vi "Write Read.vi"(5 "Byte Count":u32, 6 "Timeout ms (1000)":i32=1000, 7 "error in (no error)":errorcluster, 8 "Bytes to Write":u8[](array[numeric]), 9 "Slave Address (7-bit)":u8, 10 "I2C Ref In":T1={"myRIO Reference"={"myRIO Model"=enum."Unknown", "myRIO Hardware Reference"={"Generic FPGA Reference"=refnum, "Allow multiple opens"=FALSE}}, "I2C Channels Enum"=enum."Not Connected", "I2C Configuration"={"I2C Transfer Rate"=enum."Fast mode (400 kbps)"}}) -> (0 "error out":errorcluster, 2 "Bytes Read":u8[](array[numeric]), 3 "I2C Ref Out":T1={"myRIO Reference"={"myRIO Model"=enum."Unknown", "myRIO Hardware Reference"={"Generic FPGA Reference"=refnum, "Allow multiple opens"=FALSE}}, "I2C Channels Enum"=enum."Not Connected", "I2C Configuration"={"I2C Transfer Rate"=enum."Fast mode (400 kbps)"}})   [LabVIEW 2021, in "I2C.lvlib"]
doc: "Writes data to an Inter-Integrated Circuit (I2C) slave device and then reads a specified number of bytes of data from the I2C slave device. This VI returns the result when finishing writing or reading all the bytes, or when timing out."
uses:
  <vilib>/myRIO/Instrument Drivers/Onboard IO/I2C/I2C.lvlib
  <vilib>/myRIO/Instrument Drivers/Onboard IO/I2C/typedefs/I2C Reference.ctl
  <vilib>/myRIO/Common/Instrument Driver Framework/Utilities/typedefs/myRIO Generic Hardware Reference.ctl
  <vilib>/myRIO/Common/Instrument Driver Framework/Utilities/typedefs/Hardware Version Enum.ctl
  <vilib>/myRIO/Common/Instrument Driver Framework/Utilities/typedefs/myRIO v1.0 Reference.ctl
  <vilib>/myRIO/Common/Instrument Driver Framework/Utilities/typedefs/Generic FPGA Reference.ctl
  <vilib>/myRIO/Common/Instrument Driver Framework/myRIO v1.0/I2C/typedefs/I2C Channels Enum.ctl
  <vilib>/myRIO/Instrument Drivers/Onboard IO/I2C/typedefs/I2C Configuration.ctl
  <vilib>/myRIO/Instrument Drivers/Onboard IO/I2C/typedefs/I2C Transfer Rate.ctl
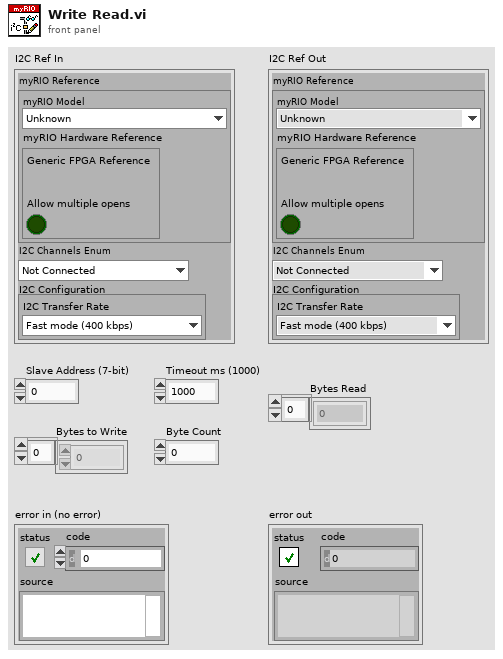
[diagram p1: front panel]
types:
  T1 = typedef "I2C.lvlib/I2C Reference.ctl" = cluster{"myRIO Reference":T2, "I2C Channels Enum":T6, "I2C Configuration":T7}
  T2 = typedef "myRIO Generic Hardware Reference.ctl" = cluster{"myRIO Model":T3, "myRIO Hardware Reference":T4}
  T3 = typedef "Hardware Version Enum.ctl" = enum16{"Unknown", "myRIO-1900", "myRIO-1950", "roboRIO", "NI ELVIS RIO CM", "ELVIS III"}
  T4 = typedef "myRIO v1.0 Reference.ctl" = cluster{"Generic FPGA Reference":T5, "Allow multiple opens":bool}
  T5 = typedef "Generic FPGA Reference.ctl" = refnum<k20>
  T6 = typedef "I2C Channels Enum.ctl" = enum16{"Not Connected", "A/I2C", "B/I2C", "I2C/I2C"}
  T7 = typedef "I2C.lvlib/I2C Configuration.ctl" = cluster{"I2C Transfer Rate":T8}
  T8 = typedef "I2C.lvlib/I2C Transfer Rate.ctl" = enum16{"Standard mode (100 kbps)", "Fast mode (400 kbps)"}
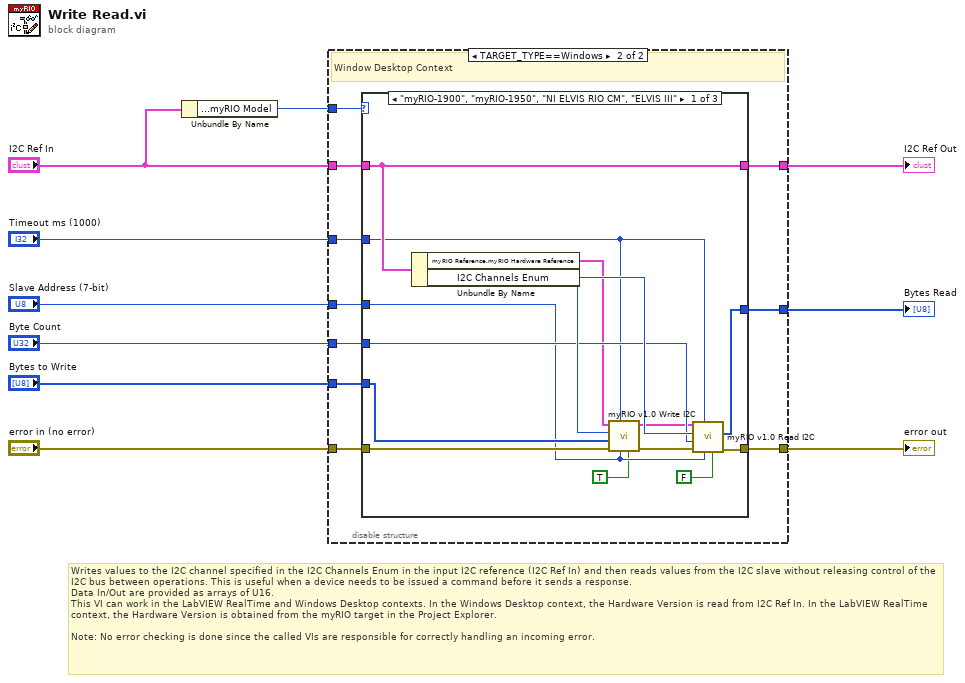
[diagram p0: block diagram]
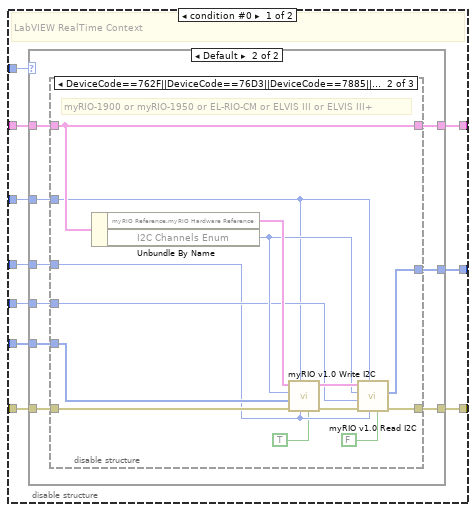
[diagram p2: hidden frame]
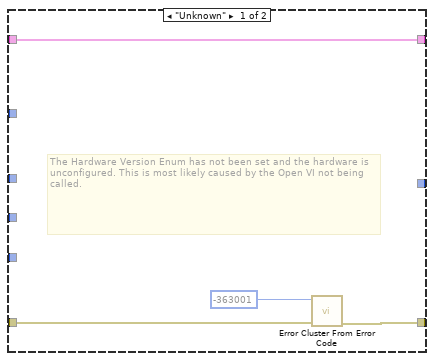
[diagram p3: hidden frame]
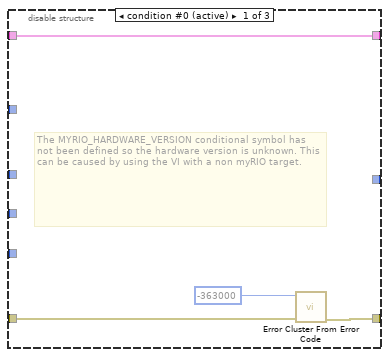
[diagram p4: hidden frame]
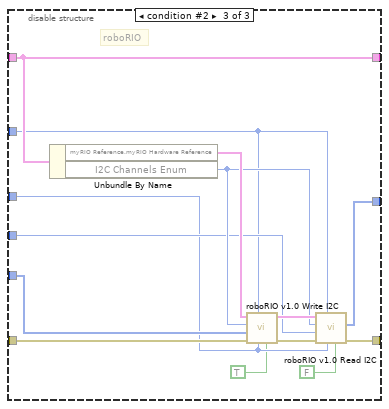
[diagram p5: hidden frame]
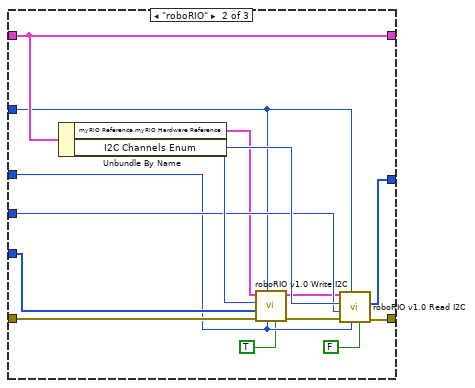
[diagram p6: hidden frame]
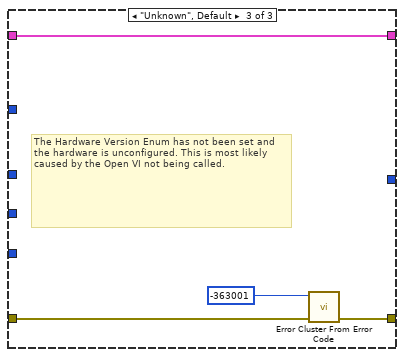
[diagram p7: hidden frame]
diagram:
  # "Writes values to the I2C channel specified in the I2C Channels Enum in the input I2C reference (I2C Ref In) and then reads values from the I2C slave without releasing control of the I2C bus between operations. This is useful when a device needs to be issued a command before it sends a response.\nData In/Out are provided as arrays of U16.\nThis VI can work in the LabVIEW RealTime and Windows Desktop contexts. In the Windows Desktop context, the Hardware Version is read from I2C Ref In. In the LabVIEW RealTime context, the Hardware Version is obtained from the myRIO target in the Project Explorer.\n\nNote: No error checking is done since the called VIs are responsible for correctly handling an incoming error."
  n1 = Unbundle By Name("I2C Ref In") -> ("myRIO Reference.myRIO Model"=w2:T3)
  n2 = disable-structure shown="TARGET_TYPE==Windows" {
    disable-tunnel: [w20 w75] -> w7
    disable-tunnel: "I2C Ref In" -> [w19 w72]
    disable-tunnel: "error in (no error)" -> [w18 w74]
    disable-tunnel: [w17 w73] -> w8
    disable-tunnel: w2 -> [w16 w71]
    disable-tunnel: "Bytes to Write" -> [w15 w70]
    disable-tunnel: "Slave Address (7-bit)" -> [w14 w69]
    disable-tunnel: "Byte Count" -> [w13 w68]
    disable-tunnel: [w12 w67] -> w3
    disable-tunnel: "Timeout ms (1000)" -> [w11 w66]
    frame condition #0 {
      # "LabVIEW RealTime Context"
      n3 = case shown="Default" w16 {
        tunnel: [w23 w33] -> w20
        tunnel: w19 -> [w21 w32]
        tunnel: w18 -> [w22 w31]
        tunnel: [w21 w30] -> w17
        tunnel: w15 -> [_ w29]
        tunnel: w14 -> [_ w28]
        tunnel: w13 -> [_ w27]
        tunnel: [_ w26] -> w12
        tunnel: w11 -> [_ w25]
        frame "Unknown" {
          # "The Hardware Version Enum has not been set and the hardware is unconfigured. This is most likely caused by the Open VI not being called."
          n4 = call <vilib>:"Error Cluster From Error Code.vi"("error in (no error)"=w22, "error code (0)"=-363001) -> ("error out"=w23:errorcluster)  [unwired: 7 in]
        }
        frame Default {
          n5 = disable-structure shown="DeviceCode==762F||DeviceCode==76D3||DeviceCode==7885||DeviceCode==7928||DeviceCode==793C" {
            disable-tunnel: w32 -> [w34 w50 w64]
            disable-tunnel: [w37 w47 w61] -> w33
            disable-tunnel: w31 -> [w35 w49 w63]
            disable-tunnel: [w34 w50 w64] -> w30
            disable-tunnel: w29 -> [_ w48 w62]
            disable-tunnel: w28 -> [_ w42 w56]
            disable-tunnel: w27 -> [_ w43 w57]
            disable-tunnel: [_ w40 w54] -> w26
            disable-tunnel: w25 -> [_ w39 w53]
            frame condition #0 (active) {
              # "The MYRIO_HARDWARE_VERSION conditional symbol has not been defined so the hardware version is unknown. This can be caused by using the VI with a non myRIO target."
              n6 = call <vilib>:"Error Cluster From Error Code.vi"("error in (no error)"=w35, "error code (0)"=-363000) -> ("error out"=w37:errorcluster)  [unwired: 7 in]
            }
            frame condition #1 {
              # "myRIO-1900 or myRIO-1950 or EL-RIO-CM or ELVIS III or ELVIS III+"
              n7 = Unbundle By Name(w50) -> ("myRIO Reference.myRIO Hardware Reference"=w51:T4, "I2C Channels Enum"=w44:T6)
              n8 = call <vilib>:"myRIO v1.0 Write I2C.vi"("Keep Bus Busy"=TRUE ("Generate STOP"), "Slave Address (7-bit)"=w42, "Timeout ms (1000)"=w39, "Error In (No Error)"=w49, "Data to Write"=w48, "Channel"=w44, "myRIO Ref In"=w51) -> ("error out"=w46:errorcluster, "myRIO Ref Out"=w45:T4)  [unwired: 3 in]
              n9 = call <vilib>:"myRIO v1.0 Read I2C.vi"("Keep Bus Busy"=FALSE, "Slave Address (7-bit)"=w42, "Timeout ms (1000)"=w39, "Error In (No Error)"=w46, "Bytes to Read"=w43, "Channel"=w44, "myRIO Ref In"=w45) -> ("error out"=w47:errorcluster, "Data Read"=w40:u8[])  [unwired: 2 in, 1 out]
            }
            frame condition #2 {
              # "roboRIO"
              n10 = Unbundle By Name(w64) -> ("myRIO Reference.myRIO Hardware Reference"=w65:T4, "I2C Channels Enum"=w58:T6)
              n11 = call <vilib>:"roboRIO v1.0 Write I2C.vi"("Keep Bus Busy"=TRUE ("Generate STOP"), "Slave Address (7-bit)"=w56, "Timeout ms (1000)"=w53, "Error In (No Error)"=w63, "Data to Write"=w62, "Channel"=w58, "myRIO Ref In"=w65) -> ("error out"=w60:errorcluster, "myRIO Ref Out"=w59:T4)  [unwired: 3 in]
              n12 = call <vilib>:"roboRIO v1.0 Read I2C.vi"("Keep Bus Busy"=FALSE, "Slave Address (7-bit)"=w56, "Timeout ms (1000)"=w53, "Error In (No Error)"=w60, "Bytes to Read"=w57, "Channel"=w58, "myRIO Ref In"=w59) -> ("error out"=w61:errorcluster, "Data Read"=w54:u8[])  [unwired: 2 in, 1 out]
            }
          }
        }
      }
    }
    frame condition #1 (active) {
      # "Window Desktop Context"
      n13 = case shown="\"myRIO-1900\", \"myRIO-1950\", \"NI ELVIS RIO CM\", \"ELVIS III\"" w71 {
        tunnel: [w80 w94 w107] -> w75
        tunnel: w72 -> [w89 w103 w104]
        tunnel: w74 -> [w88 w102 w105]
        tunnel: [w89 w103 w104] -> w73
        tunnel: w70 -> [w87 w101 _]
        tunnel: w69 -> [w79 w93 _]
        tunnel: w68 -> [w85 w99 _]
        tunnel: [w81 w95 _] -> w67
        tunnel: w66 -> [w77 w91 _]
        frame "myRIO-1900", "myRIO-1950", "NI ELVIS RIO CM", "ELVIS III" {
          n14 = Unbundle By Name(w89) -> ("myRIO Reference.myRIO Hardware Reference"=w83:T4, "I2C Channels Enum"=w86:T6)
          n15 = call <vilib>:"myRIO v1.0 Write I2C.vi"("Keep Bus Busy"=TRUE ("Generate STOP"), "Slave Address (7-bit)"=w79, "Timeout ms (1000)"=w77, "Error In (No Error)"=w88, "Data to Write"=w87, "Channel"=w86, "myRIO Ref In"=w83) -> ("error out"=w84:errorcluster, "myRIO Ref Out"=w82:T4)  [unwired: 3 in]
          n16 = call <vilib>:"myRIO v1.0 Read I2C.vi"("Keep Bus Busy"=FALSE, "Slave Address (7-bit)"=w79, "Timeout ms (1000)"=w77, "Error In (No Error)"=w84, "Bytes to Read"=w85, "Channel"=w86, "myRIO Ref In"=w82) -> ("error out"=w80:errorcluster, "Data Read"=w81:u8[])  [unwired: 2 in, 1 out]
        }
        frame "roboRIO" {
          n17 = Unbundle By Name(w103) -> ("myRIO Reference.myRIO Hardware Reference"=w97:T4, "I2C Channels Enum"=w100:T6)
          n18 = call <vilib>:"roboRIO v1.0 Write I2C.vi"("Keep Bus Busy"=TRUE ("Generate STOP"), "Slave Address (7-bit)"=w93, "Timeout ms (1000)"=w91, "Error In (No Error)"=w102, "Data to Write"=w101, "Channel"=w100, "myRIO Ref In"=w97) -> ("error out"=w98:errorcluster, "myRIO Ref Out"=w96:T4)  [unwired: 3 in]
          n19 = call <vilib>:"roboRIO v1.0 Read I2C.vi"("Keep Bus Busy"=FALSE, "Slave Address (7-bit)"=w93, "Timeout ms (1000)"=w91, "Error In (No Error)"=w98, "Bytes to Read"=w99, "Channel"=w100, "myRIO Ref In"=w96) -> ("error out"=w94:errorcluster, "Data Read"=w95:u8[])  [unwired: 2 in, 1 out]
        }
        frame "Unknown", Default {
          # "The Hardware Version Enum has not been set and the hardware is unconfigured. This is most likely caused by the Open VI not being called."
          n20 = call <vilib>:"Error Cluster From Error Code.vi"("error in (no error)"=w105, "error code (0)"=-363001) -> ("error out"=w107:errorcluster)  [unwired: 7 in]
        }
      }
    }
  }
  "I2C Ref Out" <- w8
  "error out" <- w7
  "Bytes Read" <- w3
